vi "PROJECT_Name--constant.vi"() -> (3 "PROJECT Name":string)   [LabVIEW 2022 SP3, in "Project.lvlib"]
doc: "Constant VI defining the name of the Project. This influences directory structure and other things.\n\n____\nHAMPEL SOFTWARE ENGINEERING v2.6.0 (2023-12-19 10:54)"
uses:
  Project.lvlib
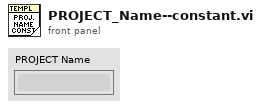
[diagram p1: front panel]
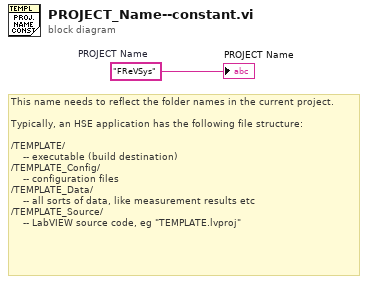
[diagram p0: block diagram]
diagram:
  w1 = "FReVSys"  # PROJECT Name
  # "This name needs to reflect the folder names in the current project.\n\nTypically, an HSE application has the following file structure:\n\n/TEMPLATE/\n    -- executable (build destination)\n/TEMPLATE_Config/\n    -- configuration files\n/TEMPLATE_Data/\n    -- all sorts of data, like measurement results etc\n/TEMPLATE_Source/\n    -- LabVIEW source code, eg \"TEMPLATE.lvproj\""
  "PROJECT Name" <- w1
